vi "TagContainer-List.vi"(8 "error in (no error)":errorcluster, 10 "with Data?(F)":bool, 11 "TagContainer":T1) -> (0 "error out":errorcluster, 1 "Data":variant[](array[variant]), 2 "names":string[](array[string]), 3 "TagContainer(dup)":T1)   [LabVIEW 2017, in "TagContainer.lvlib"]
uses:
  TagContainer.lvlib
  Typedef/TagContainer.ctl
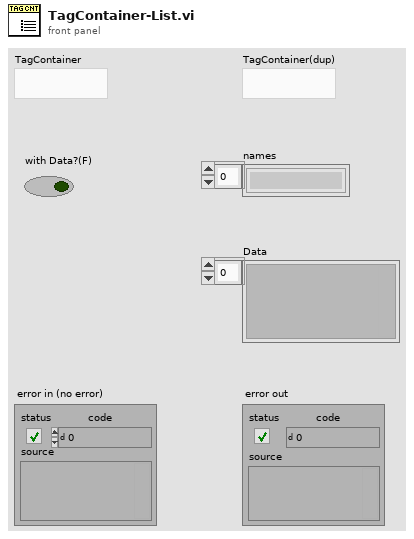
[diagram p1: front panel]
types:
  T1 = typedef "TagContainer.lvlib/TagContainer.ctl" = refnum<k1>
  T2 = typedef "TagContainer.lvlib/tagcontainer-data.ctl" = cluster{"tag-map":variant, "timestamp-map":variant, "namecacher-map":variant, "DataTypeCacher-map":variant, "Tag Adding Lock?":bool, "Global Change Timestamp":timestamp}
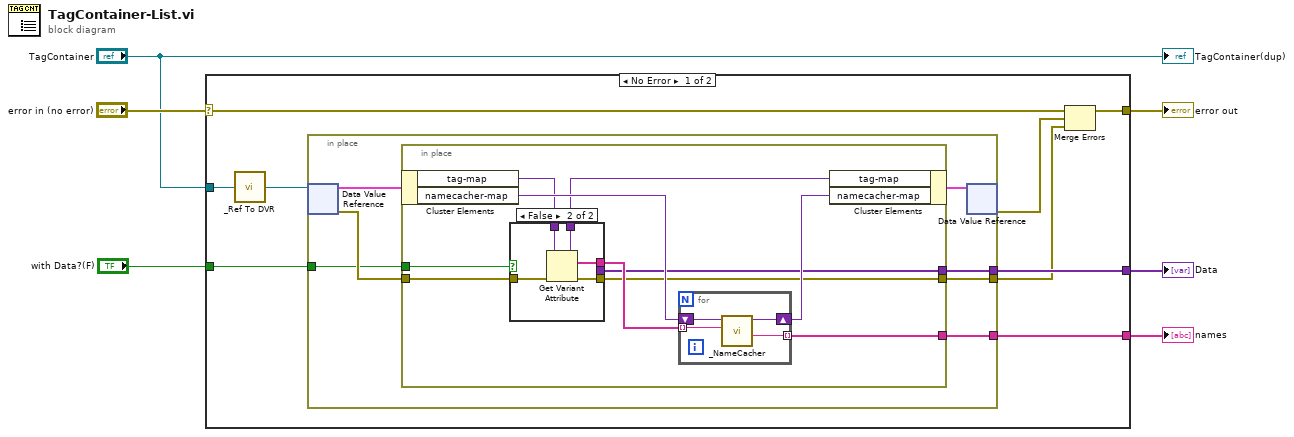
[diagram p0: block diagram]
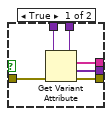
[diagram p2: hidden frame]
diagram:
  n1 = case shown="No Error" "error in (no error)" {
    selector: "error in (no error)" -> [w15 w48]
    tunnel: [w12 w48] -> w6
    tunnel: "TagContainer" -> [w14 _]
    tunnel: [w10 _] -> w3
    tunnel: [w9 _] -> w2
    tunnel: "with Data?(F)" -> [w7 _]
    frame No Error {
      n2 = call "_Ref To DVR.vi"("TagContainer"=w14) -> ("DVR"=w13:refnum<data-value>)
      n3 = in-place {
        in-place-border: [w22] -> w10
        in-place-border: [w21] -> w9
        in-place-border: [w17] -> w8
        in-place-border: w7 -> [w16]
        n4 = in-place-dvr #1(w13) -> (w20:T2, w18:errorcluster)
        n5 = in-place {
          in-place-border: [w25] -> w22
          in-place-border: [w31] -> w21
          in-place-border: w18 -> [w27]
          in-place-border: [w24] -> w17
          in-place-border: w16 -> [w23]
          n6 = in-place-cluster #2(w20) -> ("tag-map"=w29:variant, "namecacher-map"=w30:variant)
          n7 = case shown="False" w23 {
            tunnel: [w38 w43] -> w32
            tunnel: w29 -> [w37 w42]
            tunnel: [w36 w41] -> w28
            tunnel: w27 -> [w35 w40]
            tunnel: [w34 _] -> w25
            tunnel: [w33 w39] -> w24
            frame True {
              n8 = Get Variant Attribute(Variant=w37, error in=w35) -> (duplicate Variant=w36:variant, names=w38:string[], values=w34:variant[], error out=w33:errorcluster)  [unwired: 2 in]
            }
            frame False {
              n9 = Get Variant Attribute(Variant=w42, error in=w40) -> (duplicate Variant=w41:variant, names=w43:string[], error out=w39:errorcluster)  [unwired: 2 in, 1 out]
            }
          }
          n10 = for {
            tunnel: w32 -> [w47] mode=indexing
            tunnel: [w46] -> w31 mode=indexing
            shift-right: [w44] -> w26
            shift-left: w30 -> [w45]
            n11 = call "_NameCacher.vi"("key"=w47, "cacher"=w45) -> ("Raw name"=w46:string, "cacher out"=w44:variant)  [unwired: 7 in, 1 out]
          }
          n12 = in-place-cluster #2("tag-map"=w28, "namecacher-map"=w26) -> (w19:T2)
        }
        n13 = in-place-dvr #1(w19) -> (w11:errorcluster)  [unwired: 1 out]
      }
      n14 = Merge Errors(w15, w11, w8) -> (w12:errorcluster)
    }
    frame Error {
    }
  }
  "error out" <- w6
  "names" <- w2
  "Data" <- w3
  "TagContainer(dup)" <- "TagContainer"
